vi "handclear.vi"(9 "总像素":dbl, 10 "Image 3":T1) -> ()   [LabVIEW 2018]
doc: "This example shows how to compute the histogram of an image or a region in the image. This example also shows how to set up and use the display tools to select and work on different regions in the image interactively."
uses:
  <vilib>/vision/Image Controls.llb/IMAQ Image.ctl
  <vilib>/vision/NI_Vision_Development_Module.lvlib
panel:
  in  "总面积":dbl
  out "操作过程提示":string
  out "提示":string
  in  "数值":dbl min=0.0 max=2.0
  in  "恢复":bool
  out "ROI":T2
  out "大小":i32
  out "数组 2":T3(array[cluster])
  in  "删除不需要的部分":bool
  out "Image":T1(plugin-control)
  in  "Stop":bool
  # "手动剔除异常值（主要是针对火焰的总面积）"
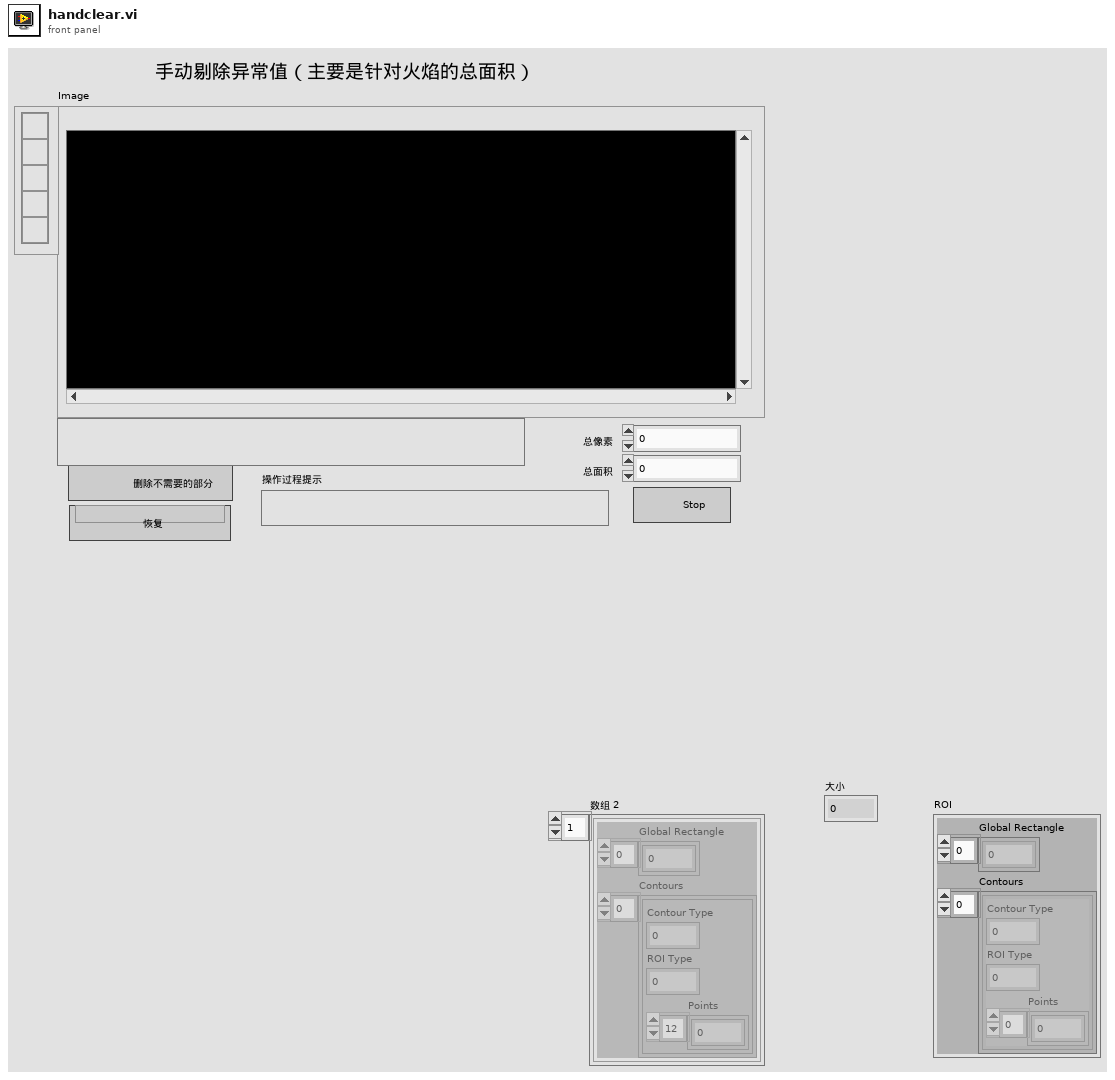
[diagram p1: front panel]
types:
  T1 = typedef "IMAQ Image.ctl" = refnum<image>
  T2 = cluster{"Global Rectangle":i32[], "Contours":cluster{"Contour Type":u32, "ROI Type":u32, "Points":i32[]}[]}
  T3 = cluster{"Global Rectangle":i32[], "Contours":cluster{"Contour Type":u32, "ROI Type":u32, "Points":i32[]}[]}[]
  T4 = typedef "Image Type" = u32
  T5 = enum8{"Enabled", "Disabled", "Disabled and Grayed Out"}
  T6 = typedef "Particle Parameters" = i32
  T7 = typedef "ROI Descriptor" = cluster{"Global Rectangle":i32[], "Contours":cluster{"ID":enum32{"External", "Internal"}, "Type":u32, "Coordinates":i32[]}[]}
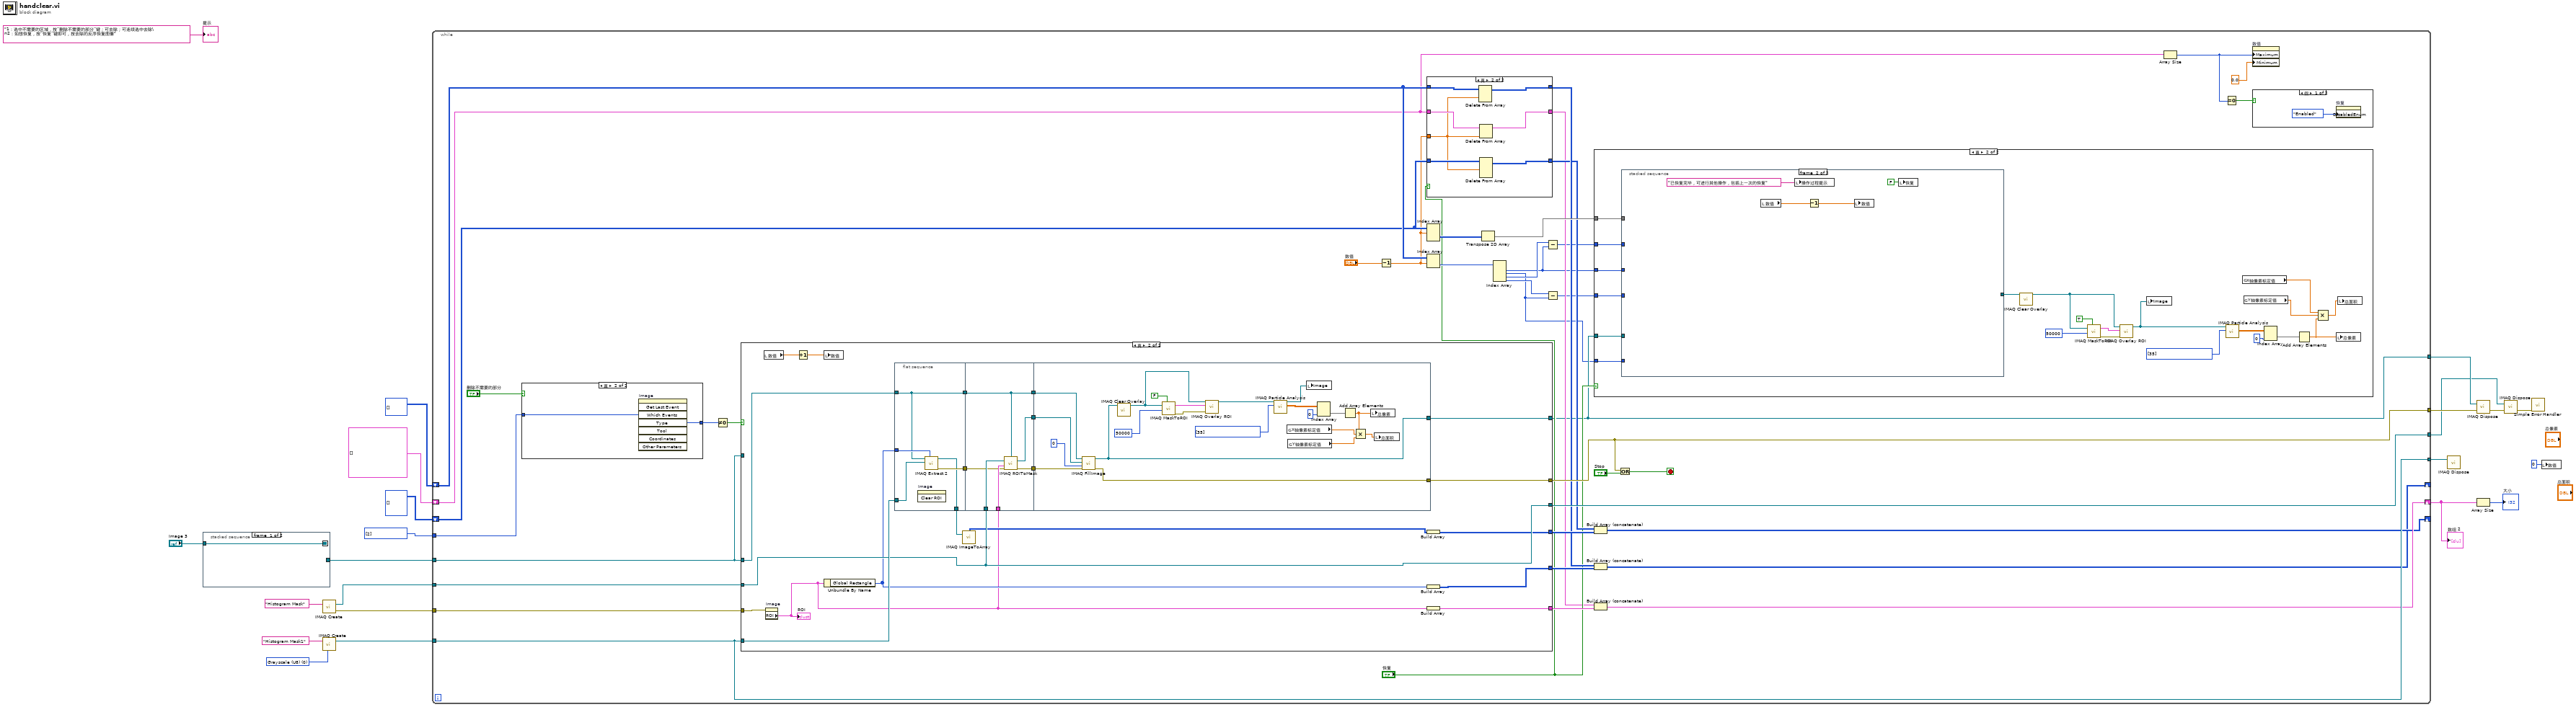
[diagram p0: block diagram]
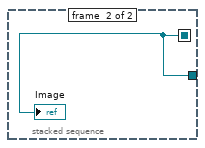
[diagram p2: hidden frame]
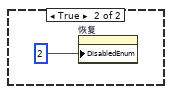
[diagram p3: hidden frame]
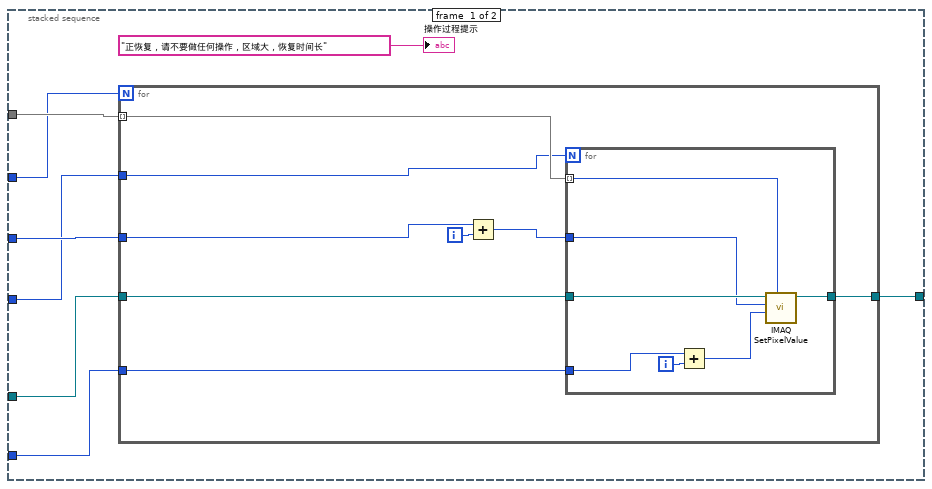
[diagram p6: hidden frame]
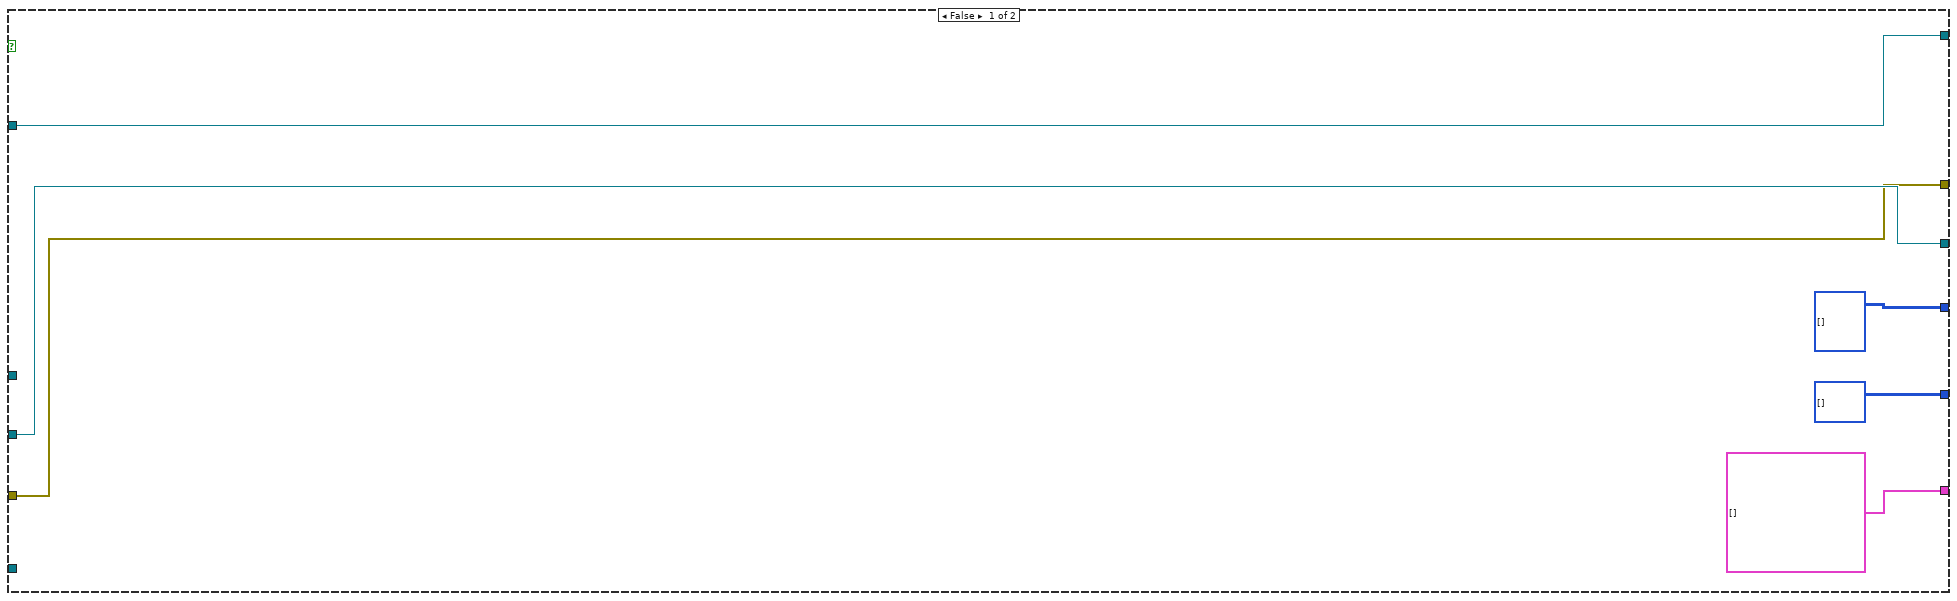
[diagram p8: hidden frame]
diagram:
  w8 = T4 0 items=["Grayscale (U8)", "Grayscale (I16)", "Grayscale (SGL)", "Complex (CSG)", "RGB (U32)", "HSL (U32)", "RGB (U64)", "Grayscale (U16)"] ("Image Type")
  w17 = i32[] [2] items=["No  event", "Click event", "Draw event", "Move event", "Size event", "Scroll event", "Activate event", "Close event", "Double click event"] ("Events list (all)")
  n1 = stacked-sequence {
    seq-local: [w23 _] -> [_ w24]
    tunnel: [_ w24] -> w3
    tunnel: "Image 3" -> [w23 _]
    frame #0 {
    }
    frame #1 {
      "Image" <- w24
    }
  }
  n2 = call "IMAQ Create"("Image Name"="Histogram Mask") -> ("New Image"=w21:T1, "error out"=w4:errorcluster)  [unwired: 4 in]
  n3 = call "IMAQ Create"("Image Name"="Histogram Mask1", "Image Type"=w8) -> ("New Image"=w13:T1)  [unwired: 3 in, 1 out]
  n4 = while {
    tunnel: w4 -> [w60]
    tunnel: w21 -> [w61]
    tunnel: [w57] -> w20
    tunnel: [w63] -> w15
    tunnel: w17 -> [w59]
    tunnel: w13 -> [w54]
    tunnel: [w54] -> w12
    shift-right: [w52] -> w11
    shift-left: T3 [] -> [w35]
    shift-right: [w42] -> _
    shift-left: i32[][][] [] -> [w39]
    shift-right: [w41] -> _
    shift-left: i32[][] [] -> [w40]
    tunnel: w3 -> [w55]
    tunnel: [w33] -> w16
    stop <- w62 stop-if-true
    n5 = case shown="真" "删除不需要的部分" {
      tunnel: w59 -> [_ w126]
      tunnel: [_ w125] -> w58
      frame False {
      }
      frame True {
        n6 = invoke on="Image" class="ImageControl" method="Get Last Event"("Which Events"=w126) -> ("Type"=w125:i32)  [unwired: 7 in, 7 out]
      }
    }
    n7 = Not Equal To 0?(x=w58) -> (x != 0?=w51:bool)
    n8 = case shown="真" w51 {
      tunnel: w55 -> [w132 _]
      tunnel: w61 -> [w131 w148]
      tunnel: [w130 w143] -> w57
      tunnel: [w131 w148] -> w63
      tunnel: [w132 w142] -> w33
      tunnel: w60 -> [w130 w152]
      tunnel: w55 -> [_ w151]
      tunnel: w54 -> [_ w150]
      tunnel: [T3 [] w136] -> w53
      tunnel: [i32[][] [] w138] -> w45
      tunnel: [i32[][][] [] w137] -> w44
      frame False {
      }
      frame True {
        n9 = local read "数值"() -> (w134:dbl)
        n10 = property on="Image" class="ImageControl"(error in=w152) -> ("ROI"=w135:T2)  [unwired: 1 in, 2 out]
        "ROI" <- w135
        n11 = Increment(x=w134) -> (x+1=w133:dbl)
        n12 = local write "数值"(w133) -> ()
        n13 = Unbundle By Name(w135) -> ("Global Rectangle"=w140:i32[])
        n14 = flat-sequence {
          tunnel: w151 -> [w155]
          tunnel: w150 -> [w157]
          tunnel: w140 -> [w156]
          tunnel: [w155] -> w149
          tunnel: [w154] -> w145
          tunnel: [w153] -> w141
          tunnel: w149 -> [w161]
          tunnel: w148 -> [w163]
          tunnel: [w162] -> w147
          tunnel: [w161] -> w146
          tunnel: w135 -> [w160]
          tunnel: w145 -> [w159]
          tunnel: [w158] -> w144
          tunnel: w147 -> [w183]
          tunnel: w146 -> [w184]
          tunnel: w144 -> [w182]
          tunnel: [w181] -> w143
          tunnel: [w175] -> w142
          frame #0 {
            n15 = invoke on="Image" class="ImageControl" method="Clear ROI"() -> ()  [unwired: 3 in, 3 out]
            n16 = call "IMAQ Extract 2"("Optional Rectangle"=w156, "Image Dst"=w157, "Image Src"=w155) -> ("error out"=w154:errorcluster, "Image Dst Out"=w153:T1)  [unwired: 7 in]
          }
          frame #1 {
            n17 = call "IMAQ ROIToMask"("error in (no error)"=w159, "ROI Descriptor"=w160, "Image"=w163, "Image Model"=w161) -> ("error out"=w158:errorcluster, "Image Out"=w162:T1)  [unwired: 2 in, 1 out]
          }
          frame #2 {
            w169 = T6[] [35] items=["Center of Mass X", "Center of Mass Y", "First Pixel X", "First Pixel Y", "Bounding Rect Left", "Bounding Rect Top", "Bounding Rect Right", "Bounding Rect Bottom", "Max Feret Diameter Start X", "Max Feret Diameter Start Y", "Max Feret Diameter End X", "Max Feret Diameter End Y", "Max Horiz. Segment Length Left", "Max Horiz. Segment Length Right", "Max Horiz. Segment Length Row", "-", "Bounding Rect Width", "Bounding Rect Height", "Bounding Rect Diagonal", "Perimeter", "Convex Hull Perimeter", "Holes' Perimeter", "Max Feret Diameter", "Equivalent Ellipse Major Axis", "Equivalent Ellipse Minor Axis", "Equivalent Ellipse Minor Axis (Feret)", "Equivalent Rect Long Side", "Equivalent Rect Short Side", "Equivalent Rect Diagonal", "Equivalent Rect Short Side (Feret)", "Average Horiz. Segment Length", "Average Vert. Segment Length", "Hydraulic Radius", "Waddel Disk Diameter", "-", "Area", "Holes' Area", "Particle & Holes' Area", "Convex Hull Area", "Image Area", "-", "Number of Holes", "Number of Horiz. Segments", "Number of Vert. Segments", "-", "Orientation", "Max Feret Diameter Orientation", "-", "% Area/Image Area", "% Area/(Particle & Holes' Area)", "Ratio of Equivalent Ellipse Axes", "Ratio of Equivalent Rect Sides", "-", "Elongation Factor", "Compactness Factor", "Heywood Circularity Factor", "Type Factor", "-", "Sum X", "Sum Y", "Sum XX", "Sum XY", "Sum YY", "Sum XXX", "Sum XXY", "Sum XYY", "Sum YYY", "-", "Moment of Inertia XX", "Moment of Inertia XY", "Moment of Inertia YY", "Moment of Inertia XXX", "Moment of Inertia XXY", "Moment of Inertia XYY", "Moment of Inertia YYY", "Norm. Moment of Inertia XX", "Norm. Moment of Inertia XY", "Norm. Moment of Inertia YY", "Norm. Moment of Inertia XXX", "Norm. Moment of Inertia XXY", "Norm. Moment of Inertia XYY", "Norm. Moment of Inertia YYY", "Hu Moment 1", "Hu Moment 2", "Hu Moment 3", "Hu Moment 4", "Hu Moment 5", "Hu Moment 6", "Hu Moment 7"] ("Pixel Measurements")
            n18 = call "IMAQ FillImage"("error in (no error)"=w182, "Pixel Value (U8, U16, I16, Float)"=0 ("Filling Value (255)"), "Image Mask"=w183, "Image"=w184) -> ("error out"=w181:errorcluster, "Image Out"=w175:T1)  [unwired: 6 in]
            n19 = call "IMAQ Clear Overlay"("Image"=w175) -> ("Image Out"=w174:T1)  [unwired: 9 in, 1 out]
            n20 = call "IMAQ MaskToROI"("External edges only (T)"=FALSE, "Image"=w174, "Max number of vectors in ROI"=50000) -> ("ROI Descriptor"=w179:T7, "error out"=w178:errorcluster)  [unwired: 4 in, 1 out]
            n21 = call "IMAQ Overlay ROI"("error in (no error)"=w178, "ROI Descriptor"=w179, "Image"=w174) -> ("Image Out"=w170:T1)  [unwired: 7 in, 1 out]
            n22 = call "IMAQ Particle Analysis"("Pixel Measurements"=w169, "Image"=w170) -> ("Particle Measurements (Pixels)"=w173:dbl[][], "Image Out (duplicate)"=w168:T1)  [unwired: 4 in, 4 out]
            n23 = global read "全局变量.vi" "X轴像素标定值"() -> (w166:dbl)
            n24 = global read "全局变量.vi" "Y轴像素标定值"() -> (w167:dbl)
            n25 = local write "Image"(w168) -> ()
            n26 = Index Array(array=w173, index (col)=0 ("禁用的索引 (列)")) -> (element=w171:dbl[])  [unwired: 1 in]
            n27 = Add Array Elements(numeric array=w171) -> (sum=w165:dbl)
            n28 = Compound Arithmetic op=MULTIPLY(w165, w166, w167) -> (w164:dbl)
            n29 = local write "总像素"(w165) -> ()
            n30 = local write "总面积"(w164) -> ()
          }
        }
        n31 = call "IMAQ ImageToArray"("Image"=w141) -> ("Image Pixels (U8)"=w139:u8[][])  [unwired: 3 in, 4 out]
        n32 = Build Array(w139) -> (w137:u8[][][])
        n33 = Build Array(w140) -> (w138:i32[][])
        n34 = Build Array(w135) -> (w136:T3)
      }
    }
    n35 = Decrement(x="数值") -> (x-1=w29:dbl)
    n36 = case shown="真" "恢复" {
      tunnel: w40 -> [w69 w76]
      tunnel: w39 -> [w68 w74]
      tunnel: [w69 w75] -> w38
      tunnel: [w68 w73] -> w37
      tunnel: w29 -> [_ w70]
      tunnel: w35 -> [w67 w72]
      tunnel: [w67 w71] -> w34
      frame False {
      }
      frame True {
        n37 = Delete From Array(array=w76, index (row)=w70) -> (array with subset deleted=w75:i32[][])  [unwired: 2 in, 1 out]
        n38 = Delete From Array(array=w72, index=w70) -> (array with subset deleted=w71:T3)  [unwired: 1 in, 1 out]
        n39 = Delete From Array(array=w74, index (dim 0)=w70) -> (array with subset deleted=w73:i32[][][])  [unwired: 3 in, 1 out]
      }
    }
    n40 = Index Array(array=w39, index (dim 0)=w29) -> (element=w47:i32[][])  [unwired: 2 in]
    n41 = Index Array(array=w40, index (row)=w29) -> (element=w48:i32[])  [unwired: 1 in]
    n42 = Transpose 2D Array(2D array=w47) -> (transposed array=w43:i32[][])
    n43 = Index Array(array=w48) -> (element #1=w25:i32, element #2=w26:i32, element #3=w50:i32, element #4=w49:i32)  [unwired: 4 in]
    n44 = Subtract(x=w50, y=w25) -> (x-y=w28:i32)
    n45 = Subtract(x=w49, y=w26) -> (x-y=w27:i32)
    n46 = case shown="真" "恢复" {
      tunnel: w33 -> [_ w97]
      tunnel: w25 -> [_ w96]
      tunnel: w26 -> [_ w95]
      tunnel: w43 -> [_ w94]
      tunnel: w28 -> [_ w93]
      tunnel: w27 -> [_ w92]
      frame False {
      }
      frame True {
        w82 = T6[] [35] items=["Center of Mass X", "Center of Mass Y", "First Pixel X", "First Pixel Y", "Bounding Rect Left", "Bounding Rect Top", "Bounding Rect Right", "Bounding Rect Bottom", "Max Feret Diameter Start X", "Max Feret Diameter Start Y", "Max Feret Diameter End X", "Max Feret Diameter End Y", "Max Horiz. Segment Length Left", "Max Horiz. Segment Length Right", "Max Horiz. Segment Length Row", "-", "Bounding Rect Width", "Bounding Rect Height", "Bounding Rect Diagonal", "Perimeter", "Convex Hull Perimeter", "Holes' Perimeter", "Max Feret Diameter", "Equivalent Ellipse Major Axis", "Equivalent Ellipse Minor Axis", "Equivalent Ellipse Minor Axis (Feret)", "Equivalent Rect Long Side", "Equivalent Rect Short Side", "Equivalent Rect Diagonal", "Equivalent Rect Short Side (Feret)", "Average Horiz. Segment Length", "Average Vert. Segment Length", "Hydraulic Radius", "Waddel Disk Diameter", "-", "Area", "Holes' Area", "Particle & Holes' Area", "Convex Hull Area", "Image Area", "-", "Number of Holes", "Number of Horiz. Segments", "Number of Vert. Segments", "-", "Orientation", "Max Feret Diameter Orientation", "-", "% Area/Image Area", "% Area/(Particle & Holes' Area)", "Ratio of Equivalent Ellipse Axes", "Ratio of Equivalent Rect Sides", "-", "Elongation Factor", "Compactness Factor", "Heywood Circularity Factor", "Type Factor", "-", "Sum X", "Sum Y", "Sum XX", "Sum XY", "Sum YY", "Sum XXX", "Sum XXY", "Sum XYY", "Sum YYY", "-", "Moment of Inertia XX", "Moment of Inertia XY", "Moment of Inertia YY", "Moment of Inertia XXX", "Moment of Inertia XXY", "Moment of Inertia XYY", "Moment of Inertia YYY", "Norm. Moment of Inertia XX", "Norm. Moment of Inertia XY", "Norm. Moment of Inertia YY", "Norm. Moment of Inertia XXX", "Norm. Moment of Inertia XXY", "Norm. Moment of Inertia XYY", "Norm. Moment of Inertia YYY", "Hu Moment 1", "Hu Moment 2", "Hu Moment 3", "Hu Moment 4", "Hu Moment 5", "Hu Moment 6", "Hu Moment 7"] ("Pixel Measurements")
        n47 = stacked-sequence {
          tunnel: w97 -> [w105 _]
          tunnel: w96 -> [w104 _]
          tunnel: w95 -> [w103 _]
          tunnel: w94 -> [w102 _]
          tunnel: w93 -> [w101 _]
          tunnel: w92 -> [w100 _]
          tunnel: [w99 _] -> w83
          frame #0 {
            n48 = for {
              N: w101 -> [_]
              tunnel: w105 -> [w113]
              tunnel: w104 -> [w111]
              tunnel: w103 -> [w109]
              tunnel: [w108] -> w99
              tunnel: w102 -> [w107] mode=indexing
              tunnel: w100 -> [w106]
              i -> [w112]
              n49 = Add(x=w111, y=w112) -> (x+y=w110:i32)
              n50 = for {
                N: w106 -> [_]
                tunnel: w113 -> [w120]
                tunnel: w110 -> [w119]
                tunnel: w109 -> [w117]
                tunnel: [w115] -> w108
                tunnel: w107 -> [w114] mode=indexing
                i -> [w118]
                n51 = Add(x=w117, y=w118) -> (x+y=w116:i32)
                n52 = call "IMAQ SetPixelValue"("Pixel Value"=w114, "Y Coordinate"=w116, "X Coordinate"=w119, "Image"=w120) -> ("Image Out"=w115:T1)  [unwired: 6 in, 1 out]
              }
            }
            "操作过程提示" <- "正恢复，请不要做任何操作，区域大，恢复时间长"
          }
          frame #1 {
            n53 = local read "数值"() -> (w123:dbl)
            n54 = local write "操作过程提示"("已恢复完毕，可进行其他操作，包括上一次的恢复" ("字符串")) -> ()
            n55 = Decrement(x=w123) -> (x-1=w122:dbl)
            n56 = local write "数值"(w122) -> ()
            n57 = local write "恢复"(FALSE ("恢复")) -> ()
          }
        }
        n58 = call "IMAQ Clear Overlay"("Image"=w83) -> ("Image Out"=w84:T1)  [unwired: 9 in, 1 out]
        n59 = call "IMAQ MaskToROI"("External edges only (T)"=TRUE, "Image"=w84, "Max number of vectors in ROI"=50000) -> ("ROI Descriptor"=w88:T7, "error out"=w87:errorcluster)  [unwired: 4 in, 1 out]
        n60 = call "IMAQ Overlay ROI"("error in (no error)"=w87, "ROI Descriptor"=w88, "Image"=w84) -> ("Image Out"=w81:T1)  [unwired: 7 in, 1 out]
        n61 = local write "Image"(w81) -> ()
        n62 = call "IMAQ Particle Analysis"("Pixel Measurements"=w82, "Image"=w81) -> ("Particle Measurements (Pixels)"=w89:dbl[][])  [unwired: 4 in, 5 out]
        n63 = global read "全局变量.vi" "X轴像素标定值"() -> (w80:dbl)
        n64 = global read "全局变量.vi" "Y轴像素标定值"() -> (w79:dbl)
        n65 = Index Array(array=w89, index (col)=0 ("禁用的索引 (列)")) -> (element=w90:dbl[])  [unwired: 1 in]
        n66 = Add Array Elements(numeric array=w90) -> (sum=w78:dbl)
        n67 = Compound Arithmetic op=MULTIPLY(w80, w79, w78) -> (w77:dbl)
        n68 = local write "总像素"(w78) -> ()
        n69 = local write "总面积"(w77) -> ()
      }
    }
    n70 = Build Array (concatenate)(w37, w44) -> (w42:i32[][][])
    n71 = Build Array (concatenate)(w38, w45) -> (w41:i32[][])
    n72 = Build Array (concatenate)(w34, w53) -> (w52:T3)
    n73 = Or(x=w57, y="Stop") -> (x .or. y?=w62:bool)
    n74 = Array Size(array=w35) -> (size(s)=w30:i32)
    n75 = Equal To 0?(x=w30) -> (x = 0?=w31:bool)
    n76 = property on="数值" class="DigNum (严格)"("Maximum"=w30, "Minimum"=0.0 ("数据输入界限:最小值")) -> ()  [unwired: 2 in, 2 out]
    n77 = case shown="假" w31 {
      frame False {
        n78 = property on="恢复" class="Bool (严格)"("DisabledEnum"=T5."Enabled" ("禁用")) -> ()  [unwired: 2 in, 2 out]
      }
      frame True {
        n79 = property on="恢复" class="Bool (严格)"("DisabledEnum"=2) -> ()  [unwired: 2 in, 2 out]
      }
    }
  }
  "数组 2" <- w11
  n80 = call "IMAQ Dispose"("Image"=w12) -> ()  [unwired: 5 in, 1 out]
  n81 = call "IMAQ Dispose"("Image"=w16, "error in (no error)"=w20) -> ("error out"=w19:errorcluster)  [unwired: 4 in]
  n82 = Array Size(array=w11) -> (size(s)=→"大小":i32)
  n83 = call "IMAQ Dispose"("Image"=w15, "error in (no error)"=w19) -> ("error out"=w18:errorcluster)  [unwired: 4 in]
  n84 = call <vilib>:"Simple Error Handler.vi"("error in (no error)"=w18) -> ()  [unwired: 4 in, 5 out]
  n85 = local write "数值"(0) -> ()
  "提示" <- "1：选中不需要的区域，按“删除不需要的部分”键；可去除；可连续选中去除\n2：如想恢复，按“恢复”键即可，按去除的反序恢复图像"
